vi "Desktop Main.vi"() -> ()   [LabVIEW 2021]
doc: "Demonstrates how to read the button value of the myRIO from the Shared Variable node."
panel:
  out "Button":bool
  out "error out":errorcluster
  in  "Stop":bool
  # "Overview: Demonstrates how to read the button value of the myRIO from the Shared Variable node.\nInstructions:\n1. Ensure RT Main.vi is already running.\n2. Run this VI. \n3. Press the user button on the myRIO device as many times as you want and observe the value changes of the Button indicator on this VI.\n4. Click Stop to stop this VI."
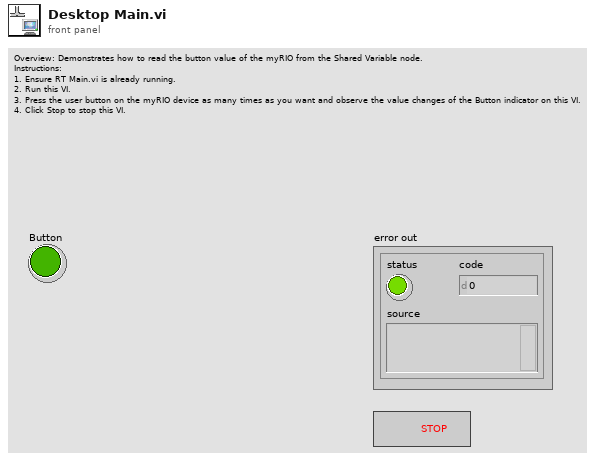
[diagram p1: front panel]
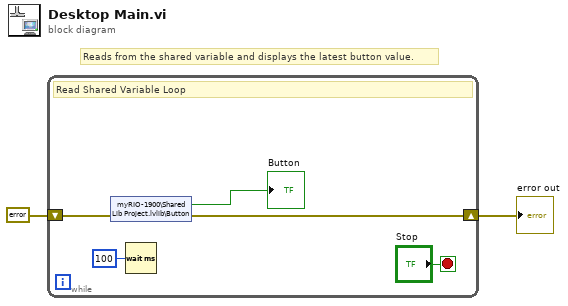
[diagram p0: block diagram]
diagram:
  # "Reads from the shared variable and displays the latest button value."
  n1 = while {
    shift-right: [w4] -> w1
    shift-left: errorcluster {"status"=FALSE, "code"=0, "source"=""} ("error in (no error)") -> [w5]
    stop <- "Stop" stop-if-true
    # "Read Shared Variable Loop"
    n2 = shared-variable "myRIO-1900\\Shared Lib Project.lvlib\\Button"(error in=w5) -> (→"Button":bool, error out=w4:errorcluster)
    n3 = Wait (ms)(milliseconds to wait=u32 100) -> ()  [unwired: 1 out]
  }
  "error out" <- w1
